vi "GetVarVal.vi"(8 "error in (no error)":errorcluster, 10 "varName":string, 11 "muExpr in":refnum<class "mupExpr.lvclass">) -> (0 "error out":errorcluster, 2 "varValue":dbl, 3 "muExpr out":refnum<class "mupExpr.lvclass">)   [LabVIEW 2015, in "mupExpr.lvclass"]
uses:
  mupExpr.lvclass
  mupExpr.lvclass/mupExpr.ctl
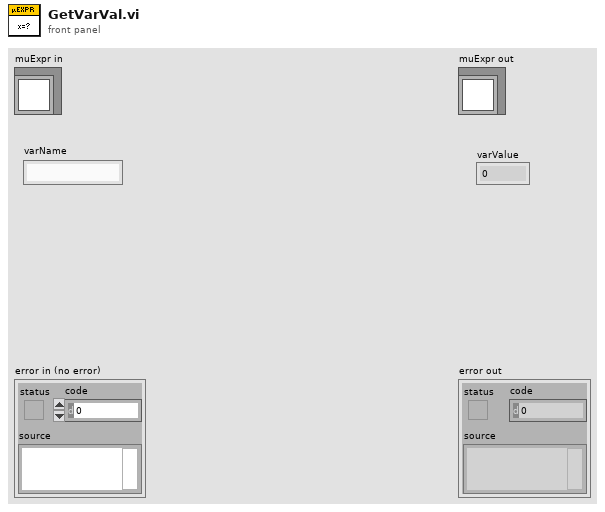
[diagram p1: front panel]
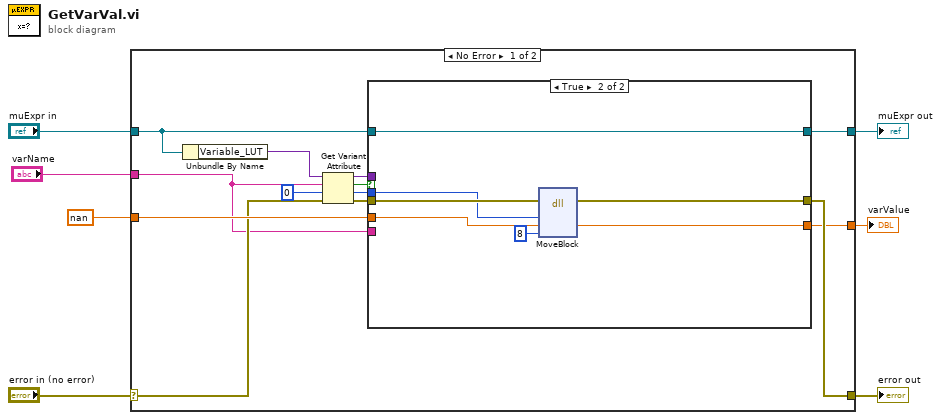
[diagram p0: block diagram]
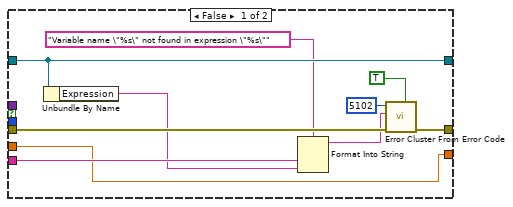
[diagram p2: hidden frame]
diagram:
  n1 = case shown="No Error" "error in (no error)" {
    selector: "error in (no error)" -> [w15 w40]
    tunnel: [w14 w40] -> w6
    tunnel: [w9 w39] -> w4
    tunnel: "muExpr in" -> [w11 w39]
    tunnel: nan ("varValue") -> [w18 w38]
    tunnel: "varName" -> [w12 _]
    tunnel: [w8 w38] -> w1
    frame No Error {
      n2 = Unbundle By Name(w11) -> ("Variable_LUT"=w20:variant)
      n3 = Get Variant Attribute(Variant=w20, name=w12, default value (empty Variant)=u64 0 ("pd"), error in=w15) -> (duplicate Variant=w10:variant, found=w13:bool, value=w16:u64, error out=w19:errorcluster)
      n4 = case shown="True" w13 {
        tunnel: w19 -> [w30 w35]
        tunnel: w18 -> [w21 w33]
        tunnel: w16 -> [_ w32]
        tunnel: [w28 w34] -> w14
        tunnel: w12 -> [w27 _]
        tunnel: w11 -> [w29 w37]
        tunnel: w10 -> [_ _]
        tunnel: [w29 w37] -> w9
        tunnel: [w21 w31] -> w8
        frame False {
          n5 = Unbundle By Name(w29) -> ("Expression"=w24:string)
          n6 = Format Into String(format string="Variable name \"%s\" not found in expression \"%s\"", w27, w24) -> (resulting string=w23:string)  [unwired: 2 in, 1 out]
          n7 = call <vilib>:"Error Cluster From Error Code.vi"("is warning? (False)"=TRUE, "error in (no error)"=w30, "error message (\"\")"=w23, "error code (0)"=5102) -> ("error out"=w28:errorcluster)  [unwired: 5 in]
        }
        frame True {
          n8 = dll-call lib="LabVIEW" fn="MoveBlock"(error in=w35, "ps"=w32, "pd"=w33, "size"=8) -> (error out=w34:errorcluster, "pd"=w31:dbl)  [unwired: 5 in, 1 out]
        }
      }
    }
    frame Error {
    }
  }
  "error out" <- w6
  "muExpr out" <- w4
  "varValue" <- w1
